vi "Save_Text_Array_to_Excel.vi"(8 "column width (1)":dbl=1.0 format="%#_13g", 9 "MS Office parameters":T1, 10 "Array":string[][](array[string]), 11 "Save Path":path) -> ()   [LabVIEW 2015]
uses:
  <vilib>/Utility/NIReport.llb/Append Text Table to Report (wrap).vi
  <vilib>/Utility/NIReport.llb/NI_report.lvclass
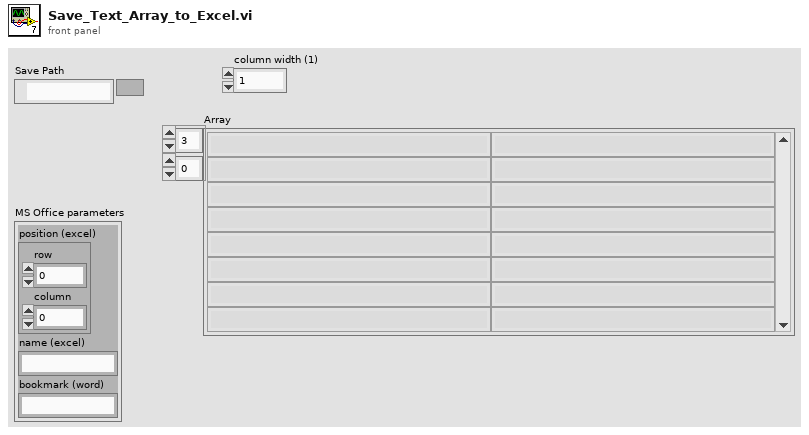
[diagram p1: front panel]
types:
  T1 = cluster{"position (excel)":cluster{"row":i32, "column":i32}, "name (excel)":string, "bookmark (word)":string}
  T2 = enum16{"maximized", "minimized", "normal", "no change"}
  T3 = enum16{"Standard Report", "HTML", "Word", "Excel"}
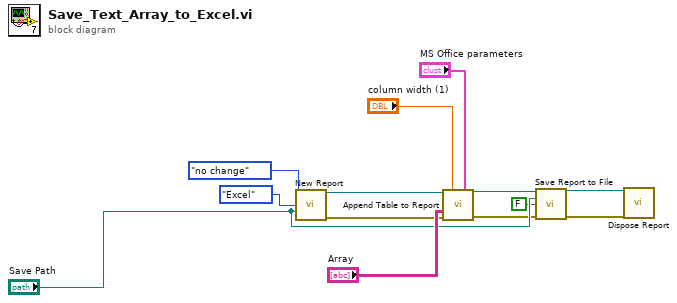
[diagram p0: block diagram]
diagram:
  n1 = call <vilib>:"New Report.vi"("window state (normal)"=T2."no change", "report type"=T3."Excel", "template (empty)"="Save Path") -> ("report out"=w4:refnum<class "NI_report.lvclass">, "error out"=w5:errorcluster)  [unwired: 11 in]
  n2 = call-poly <vilib>:"Append Table to Report.vi"("report in"=w4, "column width (1)"="column width (1)", "MS Office parameters"="MS Office parameters", "text data"="Array", "error in (no error)"=w5) -> ("report out"=w7:refnum<class "NI_report.lvclass">, "error out"=w8:errorcluster)  [unwired: 7 in, 2 out]
  n3 = call-dynamic "Save Report to File.vi"("report in"=w7, "report file path"="Save Path", "prompt to replace? (F)"=FALSE, "error in (no error)"=w8) -> ("report out"=w11:refnum<class "NI_report.lvclass">, "error out"=w12:errorcluster)  [unwired: 10 in]
  n4 = call-dynamic "Dispose Report.vi"("report in"=w11, "error in (no error)"=w12) -> ()  [unwired: 13 in, 1 out]
